vi "Set-abort.vi"(8 "error in (no error)":errorcluster, 10 "Abort":bool, 11 "Object ref in":T1) -> (0 "error out":errorcluster, 3 "Object ref out":T1)   [LabVIEW 2013, in "SLMControl.lvlib" / "SC-Main.lvclass"]
uses:
  SC-Main.lvclass
  Object-reference.ctl
  SC-Main.lvclass/SC-Main.ctl
  Read Abort.vi
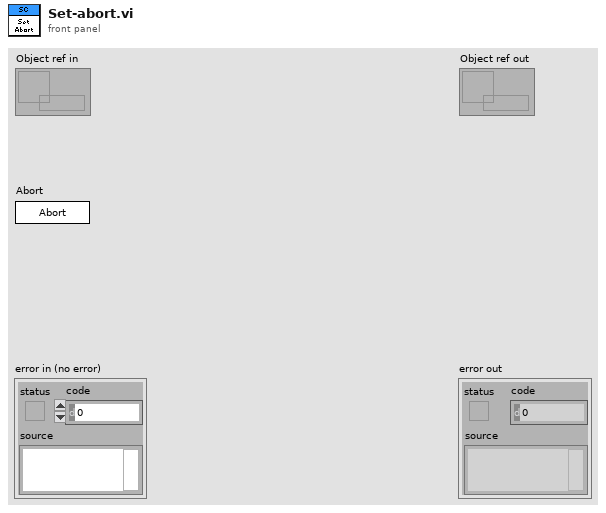
[diagram p1: front panel]
types:
  T1 = typedef "SLMControl.lvlib/SC-Main.lvclass/Object-reference.ctl" = refnum<data-value>
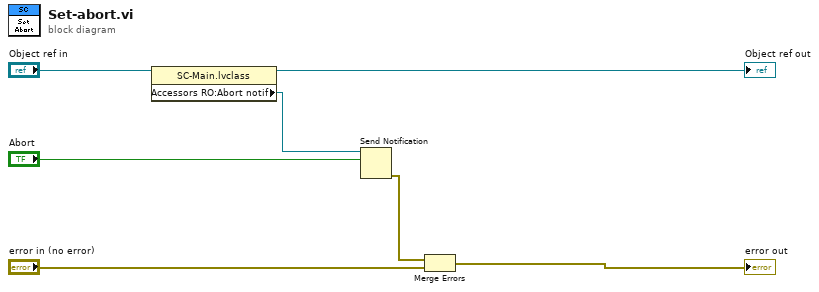
[diagram p0: block diagram]
diagram:
  n1 = property class="SC-Main.lvclass"(reference="Object ref in") -> (reference out=→"Object ref out":T1, "Accessors RO:Abort notif"=w3:refnum<notifier>)  [unwired: 1 in, 1 out]
  n2 = Send Notification(notification="Abort", notifier=w3) -> (error out=w7:errorcluster)  [unwired: 1 in, 1 out]
  n3 = Merge Errors(w7, "error in (no error)") -> (→"error out":errorcluster)
